vi "hama_orca_start.vi"(8 "error in (no error)":errorcluster {"code" format="%.0x"}, 10 "Camera ON status":bool, 11 "Camera handle in":u32) -> (0 "error out":errorcluster {"code" format="%.0x"}, 2 "Camera ON":bool=TRUE, 3 "Camera handle out":u32)   [LabVIEW 2018]
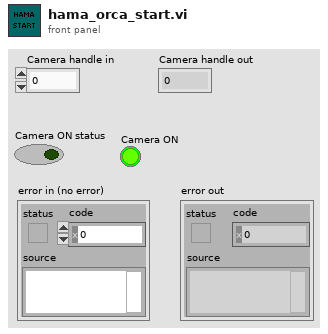
[diagram p1: front panel]
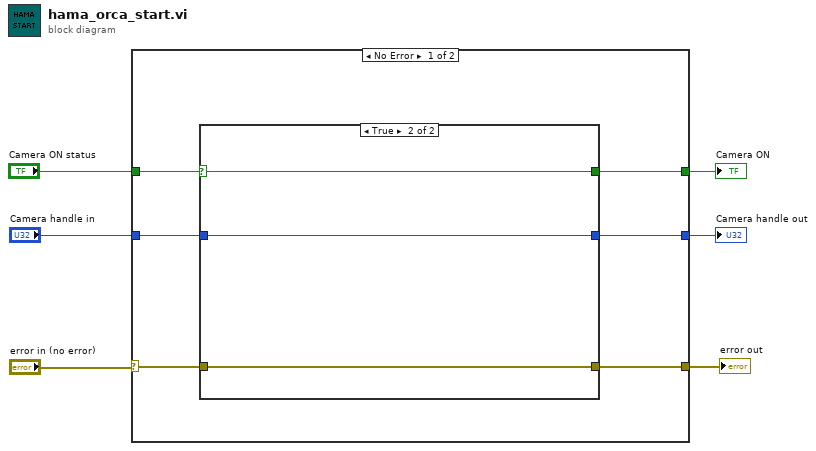
[diagram p0: block diagram]
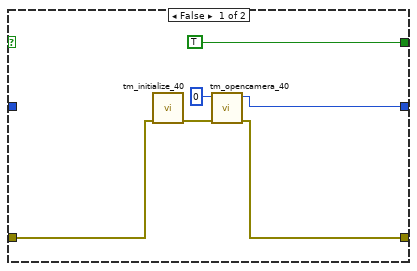
[diagram p2: hidden frame]
diagram:
  n1 = case shown="No Error" "error in (no error)" {
    selector: "error in (no error)" -> [w10 w24]
    tunnel: [w12 w24] -> w6
    tunnel: "Camera ON status" -> [w11 w23]
    tunnel: [w9 w22] -> w3
    tunnel: [w8 w23] -> w2
    tunnel: "Camera handle in" -> [w7 w22]
    frame No Error {
      n2 = case shown="True" w11 {
        selector: w11 -> [_ w21]
        tunnel: [w16 w19] -> w12
        tunnel: w10 -> [w15 w19]
        tunnel: [w14 w20] -> w9
        tunnel: [TRUE w21] -> w8
        tunnel: w7 -> [_ w20]
        frame False {
          n3 = call <userlib>:"tm_initialize_40.vi"("error in (no error)"=w15) -> ("error out"=w17:errorcluster)  [unwired: 7 in, 3 out]
          n4 = call <userlib>:"tm_opencamera_40.vi"("error in (no error)"=w17, "Camera Index"=u32 0) -> ("error out"=w16:errorcluster, "Handle out"=w14:u32)  [unwired: 7 in, 1 out]
        }
        frame True {
        }
      }
    }
    frame Error {
    }
  }
  "error out" <- w6
  "Camera handle out" <- w3
  "Camera ON" <- w2
